vi "BeamLoc.vi"(11 "BeamLoc":cluster{"X":dbl, "Y":dbl}={"X"=250.0, "Y"=250.0} {"X" min=-250.0 max=250.0; "Y" min=-250.0 max=250.0}) -> ()   [LabVIEW 2014]
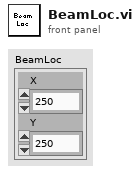
[diagram p1: front panel]
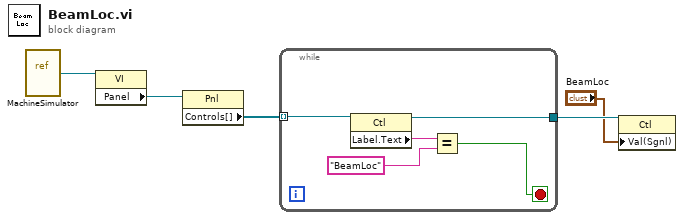
[diagram p0: block diagram]
diagram:
  n1 = vi-ref "MachineSimulator.vi"() -> (w2:refnum<vi>)
  n2 = property class="VI"(reference=w2) -> ("Panel"=w3:refnum<vi>)  [unwired: 1 in, 2 out]
  n3 = property class="Pnl"(reference=w3) -> ("Controls[]"=w5:refnum<vi>[])  [unwired: 1 in, 2 out]
  n4 = while {
    tunnel: w5 -> [w10] mode=indexing
    tunnel: [w6] -> w4
    stop <- w7 stop-if-true
    n5 = property class="Ctl"(reference=w10) -> (reference out=w6:refnum<vi>, "Label.Text"=w9:string)  [unwired: 1 in, 1 out]
    n6 = Equal?(x=w9, y="BeamLoc") -> (x = y?=w7:bool)
  }
  n7 = property class="Ctl"(reference=w4, "Val(Sgnl)"="BeamLoc") -> ()  [unwired: 1 in, 2 out]
